vi "WindDir.vi"() -> ()   [LabVIEW 2012]
panel:
  out "WindDir":dbl
  # "Overall Direction of Wind on Bay"
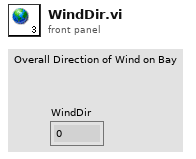
[diagram p1: front panel]
diagram:
